vi "SPD.Config Read Test01 HV_Bias.vi"(8 "Error In":errorcluster, 11 "SPD.Stand Ctrl in":T2 {"spdDeviceSession"."hidSPD.Controller"."HV_bias" format="%#_6p, V"; "spdDeviceSession"."hidSPD.Controller"."TSet" format="%#_6p, DegC"}) -> (0 "Error Out":errorcluster, 2 "HV_TestParams":T1, 3 "SPD.Stand Ctrl out":T2 {"spdDeviceSession"."hidSPD.Controller"."HV_bias" format="%#_6p, V"; "spdDeviceSession"."hidSPD.Controller"."TSet" format="%#_6p, DegC"})   [LabVIEW 2018]
uses:
  typedefs/SPD.Stand Ctrl.ctl
  Instruments/SPD HID Interface/hidSPDLibForLabView/LibVIs/hidSPD Controls/hidSPD Device Session.ctl
  Instruments/SPD HID Interface/hidSPDLibForLabView/LibVIs/hidSPD Controls/hidSPD Controller.ctl
  Instruments/KC705 DevBoard/typedefs/DevB.Session.ctl
  Instruments/KeySight 53230A/typedefs/FreqC.Session.ctl
  Instruments/KeySight 8164B/KeySight 8164B LAN InstrLib/typedefs/KeySight 8164B control.ctl
  Instruments/LeCroy SDA830/typedefs/LeCroy.Session.ctl
  typedefs/SPD.Events.ctl
  <vilib>/Utility/config.llb/Config Data RefNum.ctl
  SPDTests/SubTests/SPD.HV_Bias Test Params.vi
  <vilib>/Utility/config.llb/Read Key (I32).vi
  <vilib>/Utility/config.llb/Read Key (Double).vi
  <vilib>/Utility/config.llb/NI_LVConfig.lvlib
  Instruments/SPD HID Interface/hidSPDLibForLabView/hidSPDLibForLabView.lvlib
  Instruments/KeySight 8164B/KeySight 8164B LAN InstrLib.lvlib
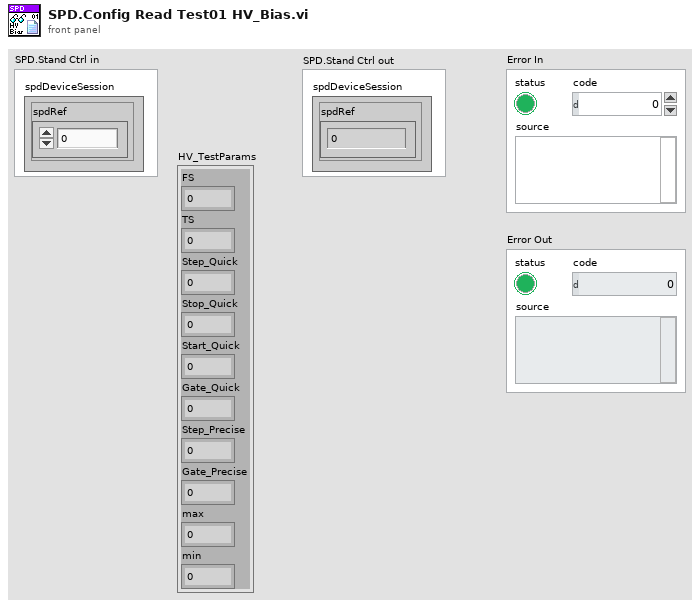
[diagram p1: front panel]
types:
  T1 = typedef "SPD.HV_Bias Test Params.vi" = cluster{"FS":i32, "TS":i32, "Step_Quick":dbl, "Stop_Quick":dbl, "Start_Quick":dbl, "Gate_Quick":dbl, "Step_Precise":dbl, "Gate_Precise":dbl, "max":dbl, "min":dbl}
  T2 = typedef "SPD.Stand Ctrl.ctl" = cluster{"spdDeviceSession":T3, "DevBSession":T5, "FreqCSession":T6, "8164BSession":T7, "LeCroySession":T8, "Events":T9, "configFile":T10}
  T3 = typedef "hidSPDLibForLabView.lvlib/hidSPD Device Session.ctl" = cluster{"spdRef":u64, "connected":bool, "spdName":string, "hidSPD.Controller":T4}
  T4 = typedef "hidSPDLibForLabView.lvlib/hidSPD Controller.ctl" = cluster{"TSet":sgl, "HV_bias":sgl, "DDS_stb_code":u16}
  T5 = typedef "DevB.Session.ctl" = cluster{"DevBRef":refnum<visa-resource-name>, "connected":bool}
  T6 = typedef "FreqC.Session.ctl" = cluster{"FreqCRef":refnum<visa-resource-name>, "timeout":dbl, "connected":bool}
  T7 = typedef "KeySight 8164B LAN InstrLib.lvlib/KeySight 8164B control.ctl" = cluster{"Connection ID":refnum<k5>, "Connected":bool, "Info":string, "Slots Info":string[]}
  T8 = typedef "LeCroy.Session.ctl" = cluster{"LeCroySession":refnum<visa-resource-name>, "connected":bool}
  T9 = typedef "SPD.Events.ctl" = cluster{"DCRTest":refnum<user-event>, "Stop":refnum<user-event>}
  T10 = typedef "NI_LVConfig.lvlib/Config Data RefNum.ctl" = refnum<k1>
  T11 = cluster{"value":i32, "value":i32, "value":dbl, "value":dbl, "value":dbl, "value":dbl, "value":dbl, "value":dbl, "value":dbl, "value":dbl}
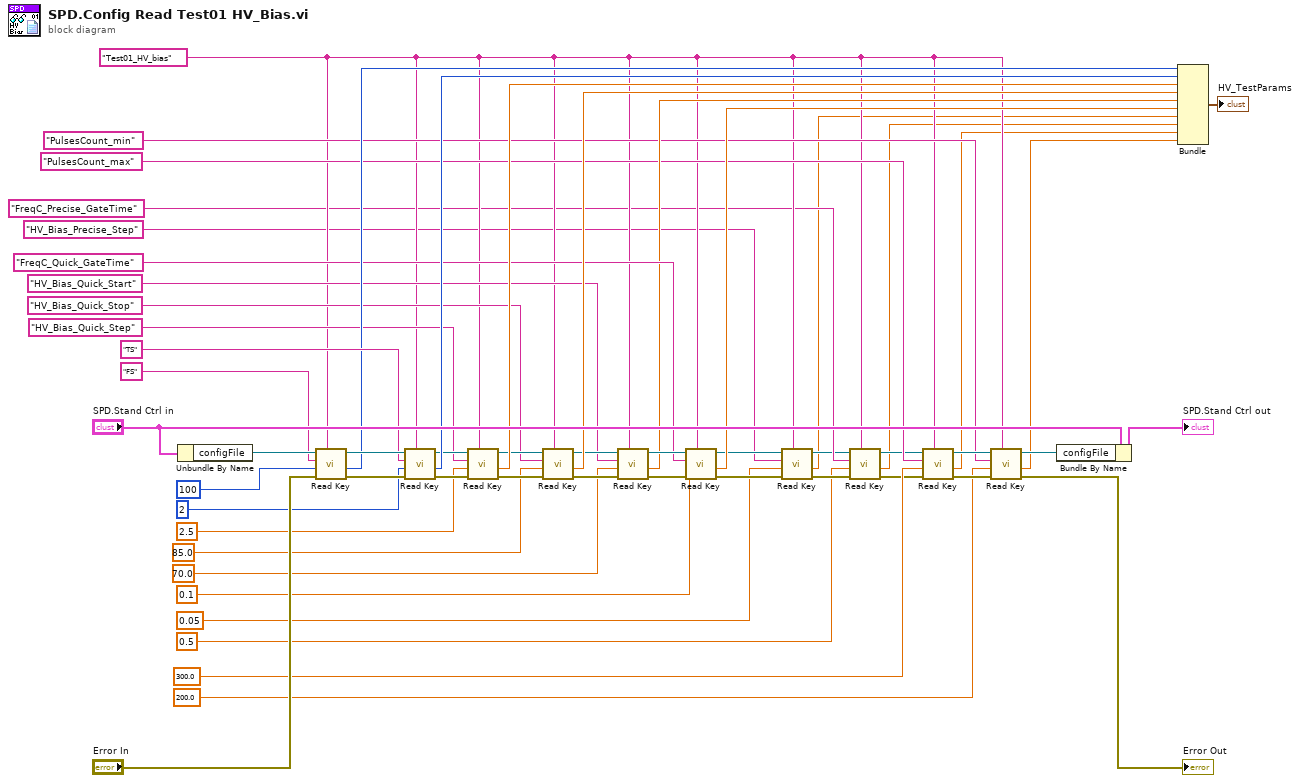
[diagram p0: block diagram]
diagram:
  w13 = "Test01_HV_bias" ("section")
  n1 = Unbundle By Name("SPD.Stand Ctrl in") -> ("configFile"=w54:T10)
  n2 = call-poly <vilib>:"Read Key.vi"("section"=w13, "error in (no error)"="Error In", "default value"=100, "key"="FS", "refnum"=w54) -> ("error out"=w50:errorcluster, "value"=w46:i32, "refnum out"=w49:T10)  [unwired: 3 in, 1 out]
  n3 = call-poly <vilib>:"Read Key.vi"("section"=w13, "error in (no error)"=w50, "default value"=2, "key"="TS", "refnum"=w49) -> ("error out"=w43:errorcluster, "value"=w45:i32, "refnum out"=w44:T10)  [unwired: 3 in, 1 out]
  n4 = call-poly <vilib>:"Read Key.vi"("section"=w13, "error in (no error)"=w43, "default value"=2.5, "key"="HV_Bias_Quick_Step", "refnum"=w44) -> ("error out"=w38:errorcluster, "value"=w40:dbl, "refnum out"=w39:T10)  [unwired: 3 in, 1 out]
  n5 = call-poly <vilib>:"Read Key.vi"("section"=w13, "error in (no error)"=w38, "default value"=85.0, "key"="HV_Bias_Quick_Stop", "refnum"=w39) -> ("error out"=w33:errorcluster, "value"=w35:dbl, "refnum out"=w34:T10)  [unwired: 3 in, 1 out]
  n6 = call-poly <vilib>:"Read Key.vi"("section"=w13, "error in (no error)"=w33, "default value"=70.0, "key"="HV_Bias_Quick_Start", "refnum"=w34) -> ("error out"=w26:errorcluster, "value"=w28:dbl, "refnum out"=w30:T10)  [unwired: 3 in, 1 out]
  n7 = call-poly <vilib>:"Read Key.vi"("section"=w13, "error in (no error)"=w26, "default value"=0.1, "key"="FreqC_Quick_GateTime", "refnum"=w30) -> ("error out"=w14:errorcluster, "value"=w25:dbl, "refnum out"=w15:T10)  [unwired: 3 in, 1 out]
  n8 = call-poly <vilib>:"Read Key.vi"("section"=w13, "error in (no error)"=w14, "default value"=0.05, "key"="HV_Bias_Precise_Step", "refnum"=w15) -> ("error out"=w16:errorcluster, "value"=w5:dbl, "refnum out"=w8:T10)  [unwired: 3 in, 1 out]
  n9 = call-poly <vilib>:"Read Key.vi"("section"=w13, "error in (no error)"=w16, "default value"=0.5, "key"="FreqC_Precise_GateTime", "refnum"=w8) -> ("error out"=w6:errorcluster, "value"=w4:dbl, "refnum out"=w7:T10)  [unwired: 3 in, 1 out]
  n10 = call-poly <vilib>:"Read Key.vi"("section"=w13, "error in (no error)"=w6, "default value"=300.0, "key"="PulsesCount_max", "refnum"=w7) -> ("error out"=w22:errorcluster, "value"=w3:dbl, "refnum out"=w24:T10)  [unwired: 3 in, 1 out]
  n11 = call-poly <vilib>:"Read Key.vi"("section"=w13, "error in (no error)"=w22, "default value"=200.0, "key"="PulsesCount_min", "refnum"=w24) -> ("error out"=→"Error Out":errorcluster, "value"=w2:dbl, "refnum out"=w23:T10)  [unwired: 3 in, 1 out]
  n12 = Bundle By Name(cluster="SPD.Stand Ctrl in", "configFile"=w23) -> (→"SPD.Stand Ctrl out":T2)
  n13 = Bundle("value"=w46, "value"=w45, "value"=w40, "value"=w35, "value"=w28, "value"=w25, "value"=w5, "value"=w4, "value"=w3, "value"=w2) -> (→"HV_TestParams":T11)  [unwired: 1 in]
